vi "DAC Configure FP View.vi"(8 "error in":errorcluster, 11 "DAC TEG Temp in":refnum<class "DAC TEG Temp.lvclass">) -> (0 "error out":errorcluster, 3 "DAC TEG Temp out":refnum<class "DAC TEG Temp.lvclass">)   [LabVIEW 2019, in "DAC.lvlib" / "DAC TEG Temp.lvclass"]
uses:
  DAC TEG Temp.lvclass
  Results/Results Method.ctl
  Results/Heat Flow Results/Heat Flow Results.lvclass
  DAC TEG Temp.lvclass/DAC TEG Temp.ctl
  Results/Heat Flow Results/Heat Flow Results.lvclass/Heat Flow Results.ctl
  Results/Results.lvlib
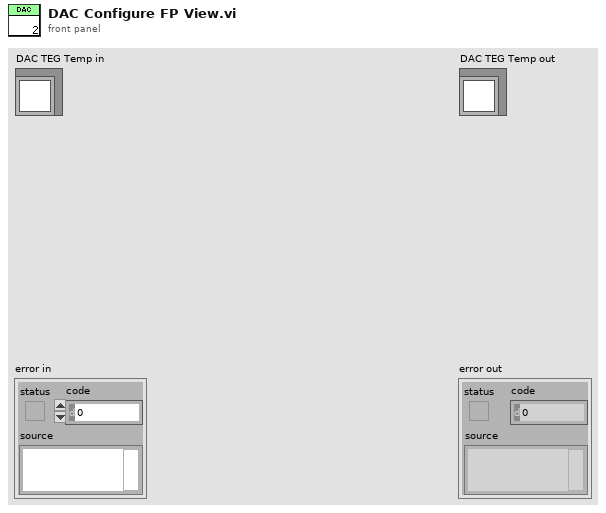
[diagram p1: front panel]
types:
  T1 = typedef "Results.lvlib/Results Method.ctl" = enum16{"Get", "Set"}
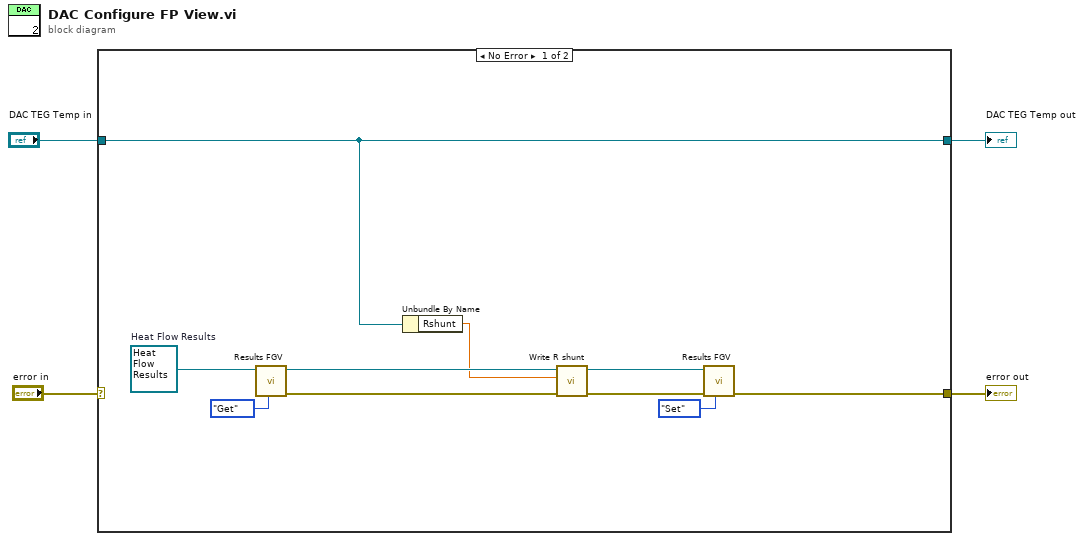
[diagram p0: block diagram]
diagram:
  n1 = case shown="No Error" "error in" {
    selector: "error in" -> [_ w16]
    tunnel: [w14 w16] -> w1
    tunnel: [w11 w15] -> w2
    tunnel: "DAC TEG Temp in" -> [w11 w15]
    frame No Error {
      w10 = refnum<class "Heat Flow Results.lvclass"> refnum  # Heat Flow Results
      n2 = call-dynamic "Results FGV.vi"("Method"=Results_Method."Get", "Results in"=w10) -> ("error out"=w6:errorcluster, "Results out"=w9:refnum<class "Heat Flow Results.lvclass">)  [unwired: 8 in]
      n3 = Unbundle By Name(w11) -> ("Rshunt"=w7:dbl)
      n4 = call "Write R shunt.vi"("error in (no error)"=w6, "R shunt"=w7, "Heat Flow Results in"=w9) -> ("error out"=w5:errorcluster, "Heat Flow Results out"=w8:refnum<class "Heat Flow Results.lvclass">)  [unwired: 7 in]
      n5 = call-dynamic "Results FGV.vi"("Method"=Results_Method."Set", "error in"=w5, "Results in"=w8) -> ("error out"=w14:errorcluster)  [unwired: 7 in, 1 out]
    }
    frame Error {
    }
  }
  "error out" <- w1
  "DAC TEG Temp out" <- w2
